vi "xyz_movematrix.vi"(4 "z":dbl(slide) scale=-3.14..3.14, 5 "y":dbl(slide) scale=-3.14..3.14, 6 "x":dbl(slide) scale=-3.14..3.14, 7 "matrix in":dbl[][](array[numeric])=[[1.0, 0.0, 0.0, 0.0], [0.0, 1.0, 0.0, 0.0], [0.0, 0.0, 1.0, 0.0], [0.0, 0.0, 0.0, 1.0]]) -> (3 "matrix out":dbl[][](array[numeric]))   [LabVIEW 2017]
uses:
  <vilib>/Analysis/baseanly.llb/Real A x B.vi
  <vilib>/Analysis/NI_AALBase.lvlib
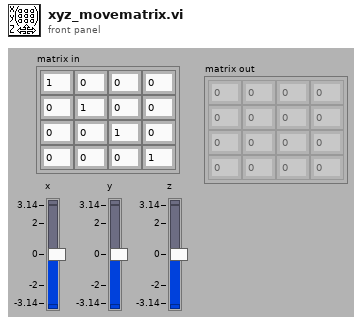
[diagram p1: front panel]
types:
  T1 = typedef "NI_Matrix.lvlib/RealMatrix.ctl" = dbl[][]
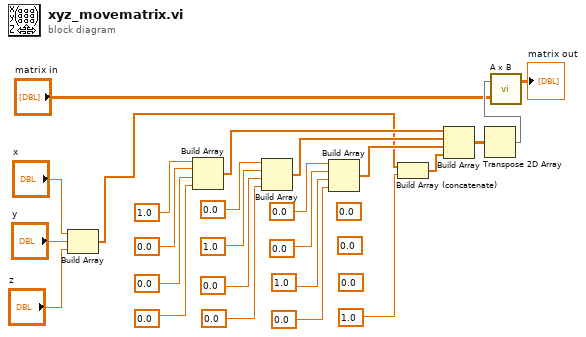
[diagram p0: block diagram]
diagram:
  (unwired) 0.0
  (unwired) 0.0
  (unwired) 0.0
  n1 = Build Array("x", "y", "z") -> (w4:dbl[])
  n2 = Build Array(1.0, 0.0, 0.0, 0.0) -> (w10:dbl[])
  n3 = Build Array(0.0, 1.0, 0.0, 0.0) -> (w9:dbl[])
  n4 = Build Array(0.0, 0.0, 1.0, 0.0) -> (w8:dbl[])
  n5 = Build Array (concatenate)(w4, 1.0) -> (w13:dbl[])
  n6 = Build Array(w10, w9, w8, w13) -> (w23:dbl[][])
  n7 = Transpose 2D Array(2D array=w23) -> (transposed array=w2:dbl[][])
  n8 = call-poly <vilib>:"A x B.vi"("B"="matrix in", "A"=w2) -> ("A x B"=→"matrix out":T1)  [unwired: 1 out]
